vi "DAQ-node.vi"() -> ()   [LabVIEW 2024]
uses:
  CTRsample/Control/StreamTypeDef.ctl
  CTRsample/Control/streamIO_states.ctl
  <vilib>/Platform/TimedLoop/XDataNode/timing_clust.ctl
  <vilib>/Platform/TimedLoop/XDataNode/nitl_modes.ctl
  <vilib>/Platform/TimedLoop/XDataNode/wakeup.ctl
  <vilib>/DAQmx/read.llb/DAQmx Read (Analog 2D DBL NChan NSamp).vi
  <vilib>/DAQmx/create/channels.llb/DAQmx Create Channel (AI-Voltage-Basic).vi
  <vilib>/DAQmx/configure/timing.llb/DAQmx Timing (Sample Clock).vi
  Control/state.vi
  <vilib>/DAQmx/miscellaneous.llb/DAQmx Fill In Error Info.vi
  <vilib>/platform/TimedLoop/XDataNode/XDataNode.xnode
  <vilib>/Platform/TimedLoop/XDataNode/XDNodeRunTimeDep.lvlib
panel:
  out "dT":i64
  out "Clock (ms)":cluster{i64, "Period":i64}(graph)
  out "error out":errorcluster
  in  "StreamTypeDef":T1
  out "Waveform Chart":dbl[][](graph)
  in  "stop":bool
  in  "error in":errorcluster
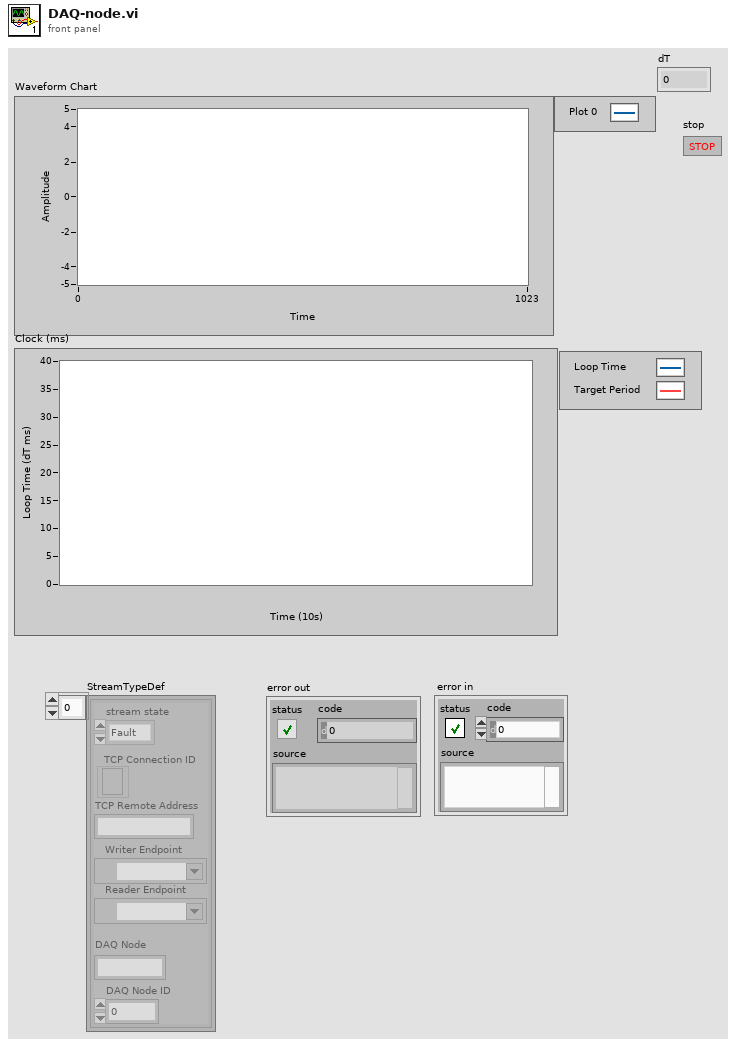
[diagram p1: front panel]
types:
  T1 = typedef "StreamTypeDef.ctl" = cluster{"stream state":T2, "TCP Remote Address":string, "TCP Connection ID":refnum<k5>, "DAQ Node":string, "DAQ Node ID":i32, "Writer Endpoint":refnum<k21>, "Reader Endpoint":refnum<k21>}[]
  T2 = typedef "streamIO_states.ctl" = enum16{"Fault", "Initilize", "Stream", "Close"}
  T3 = cluster{"StreamTypeDef[0]":cluster{"stream state":T2, "TCP Remote Address":string, "TCP Connection ID":refnum<k5>, "DAQ Node":string, "DAQ Node ID":i32, "Writer Endpoint":refnum<k21>, "Reader Endpoint":refnum<k21>}}
  T4 = cluster{"stream state":T2, "TCP Remote Address":string, "TCP Connection ID":refnum<k5>, "DAQ Node":string, "DAQ Node ID":i32, "Writer Endpoint":refnum<k21>, "Reader Endpoint":refnum<k21>}
  T5 = typedef "XDNodeRunTimeDep.lvlib/timing_clust.ctl" = cluster{"Expected End [f-1]":u64, "Actual End [f-1]":u64, "Finished Late? [f-1]":bool, "Expected End [i-1]":u64, "Actual End [i-1]":u64, "Finished Late? [i-1]":bool, "Expected Start [i]":u64, "Actual Start [i]":u64, "Expected Start [f]":u64, "Actual Start [f]":u64, "Source Name":string, "Structure Name":string, "Period":i64, "Deadline":i64, "Offset":i64, "Start":i64, "Priority":i32, "Timeout":i32, "Mode":T6, "Wakeup Reason":T7, "Error":errorcluster, "Source Type":string, "Secondary Source Type":string, "Global End Time":u64, "Global Start Time":u64, "Frame Duration":u64, "Iteration Duration":u64, "Assigned CPU":i32, "I/O Scan Engine Mode":u32}
  T6 = typedef "XDNodeRunTimeDep.lvlib/nitl_modes.ctl" = enum32{"No Change", "Process missed periods, maintain original phase", "Discard missed periods, maintain original phase", "Process missed periods, ignore original phase", "Discard missed periods, ignore original phase"}
  T7 = typedef "XDNodeRunTimeDep.lvlib/wakeup.ctl" = enum32{"Normal", "Aborted", "Asynchronous wakeup", "Timing source error", "Timed loop error", "Timeout"}
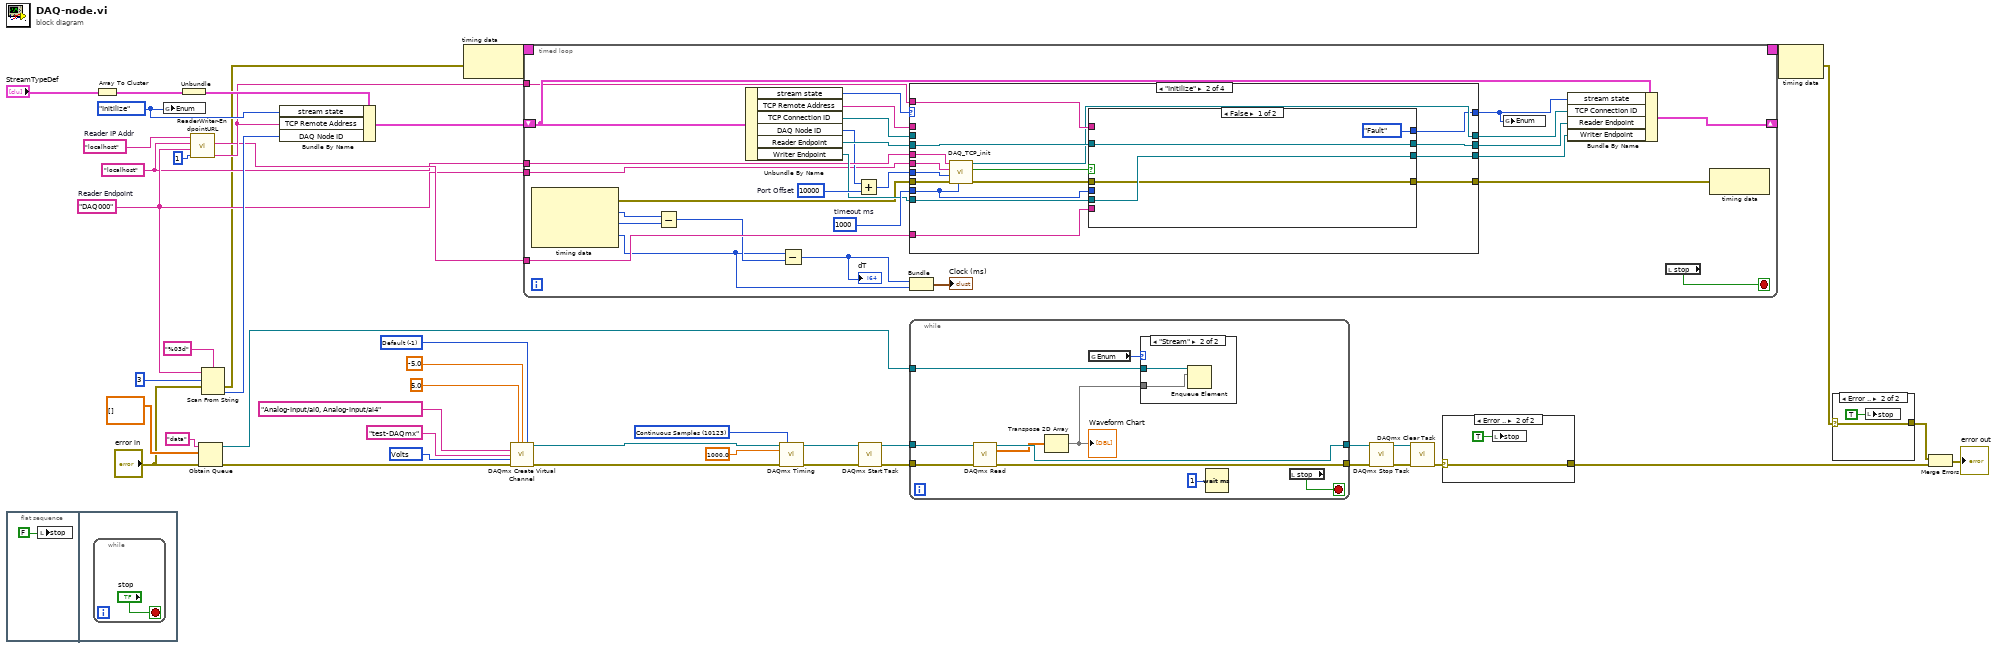
[diagram p0: block diagram]
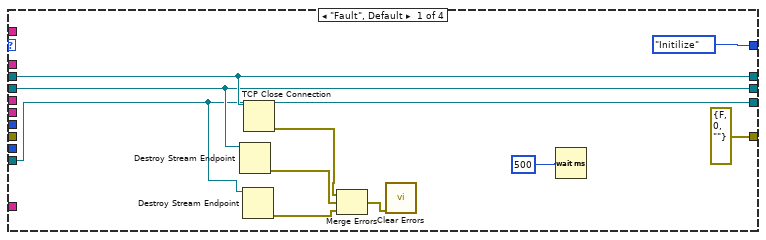
[diagram p4: hidden frame]
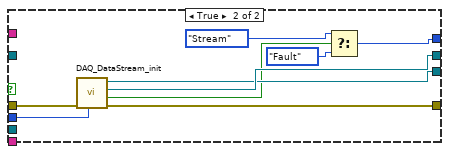
[diagram p5: hidden frame]
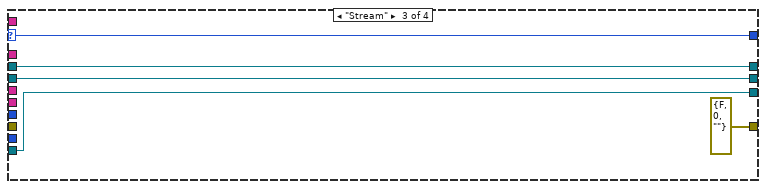
[diagram p6: hidden frame]
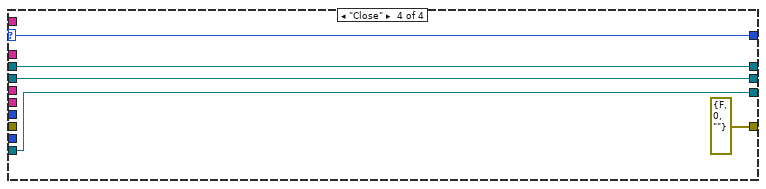
[diagram p7: hidden frame]
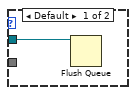
[diagram p8: hidden frame]
diagram:
  w11 = "localhost" ("DAQ IR Addr")
  w15 = "localhost"  # Reader IP Addr
  w12 = "DAQ000"  # Reader Endpoint
  w20 = streamIO_states."Initilize" ("Enum")
  w35 = 10123 items=["Finite Samples"=10178, "Continuous Samples"=10123, "Hardware Timed Single Point"=12522] ("sample mode")
  w38 = 10348 items=["Volts"=10348, "From Custom Scale"=10065] ("units")
  w43 = -1 items=["Default"=-1, "RSE"=10083, "NRSE"=10078, "Differential"=10106, "Pseudodifferential"=12529] ("input terminal configuration")
  n1 = flat-sequence {
    frame #0 {
      n2 = local write "stop"(FALSE ("stop")) -> ()
    }
    frame #1 {
      n3 = while {
        stop <- "stop" stop-if-true
      }
    }
  }
  n4 = Array To Cluster(array="StreamTypeDef") -> (cluster=w23:T3)
  n5 = global write "state.vi" "Enum"(w20) -> ()
  n6 = Unbundle(w23) -> ("StreamTypeDef[0]"=w22:T4)
  n7 = call "ReaderWriter-EndpointURL.vi"("CTR ID #"=1 ("DAQ ID #"), "DAQ Endpoint"=w12, "CTR IR Addr"=w11, "DAQ IP Addr"=w15) -> ("DAQ Endpoint"=w14:string, "CTR URL"=w13:string)  [unwired: 4 in, 2 out]
  n8 = Obtain Queue(name (unnamed)="data", element data type=dbl[][] [] ("data"), error in (no error)="error in") -> (queue out=w25:refnum<queue>, error out=w8:errorcluster)  [unwired: 2 in, 1 out]
  n9 = Scan From String(format string="%03d", input string=w12, initial scan location=u32 3, error in="error in") -> (error out=w6:errorcluster, output 1=w17:i32)  [unwired: 1 in, 2 out]
  n10 = Bundle By Name(cluster=w22, "stream state"=w20, "TCP Remote Address"=w14, "DAQ Node ID"=w17) -> (w21:T4)
  n11 = node-c288(w6) -> (w10:T5)
  n12 = call-poly <vilib>:"DAQmx Create Virtual Channel.vi"("maximum value"=5.0, "minimum value"=-5.0, "input terminal configuration"=w43, "physical channels"=tag "Analog-Input/ai0, Analog-Input/ai4", "name to assign"="test-DAQmx", "units"=w38, "error in"=w8) -> ("task out"=w34:refnum<k21>, "error out"=w28:errorcluster)  [unwired: 7 in]
  n13 = timed-loop {
    shift-right: [w73] -> _
    shift-left: w21 -> [w72]
    tunnel: w11 -> [w62]
    tunnel: w12 -> [w60]
    tunnel: w14 -> [w59]
    tunnel: w13 -> [w58]
    timing: w10 -> [_]
    timing-out: [_] -> w9
    stop <- w75 stop-if-true
    w66 = 1000  # timeout ms
    w68 = 10000  # Port Offset
    n14 = node-c288() -> (w55:errorcluster, w52:i64, w51:i64, w49:i64)  [unwired: 1 in]
    n15 = Subtract(x=w52, y=w51) -> (x-y=w50:i64)
    n16 = Unbundle By Name(w72) -> ("stream state"=w74:T2, "TCP Remote Address"=w70:string, "TCP Connection ID"=w69:refnum<k5>, "DAQ Node ID"=w61:i32, "Reader Endpoint"=w65:refnum<k21>, "Writer Endpoint"=w64:refnum<k21>)
    n17 = Subtract(x=w49, y=w50) -> (x-y=w48:i64)
    "dT" <- w48
    n18 = Add(x=w61, y=w68) -> (x+y=w67:i32)
    n19 = case shown="\"Initilize\"" w74 {
      selector: w74 -> [_ _ w127 w132]
      tunnel: [streamIO_states."Initilize" ("Enum") w94 w127 w132] -> w71
      tunnel: w70 -> [_ _ _ _]
      tunnel: w69 -> [w88 _ w125 w131]
      tunnel: w67 -> [_ w103 _ _]
      tunnel: w66 -> [_ w100 _ _]
      tunnel: w65 -> [w87 w104 w124 w130]
      tunnel: w64 -> [w86 w105 w123 w129]
      tunnel: [w88 w99 w125 w131] -> w63
      tunnel: w62 -> [_ w98 _ _]
      tunnel: w60 -> [_ w97 _ _]
      tunnel: w59 -> [_ w109 _ _]
      tunnel: w58 -> [_ w108 _ _]
      tunnel: [w86 w107 w123 w129] -> w56
      tunnel: [w87 w106 w124 w130] -> w57
      tunnel: [errorcluster {"status"=FALSE, "code"=0, "source"=""} ("error out") w96 errorcluster {"status"=FALSE, "code"=0, "source"=""} ("error out") errorcluster {"status"=FALSE, "code"=0, "source"=""} ("error out")] -> w54
      tunnel: w55 -> [_ w95 _ _]
      frame "Fault", Default {
        n20 = Destroy Stream Endpoint(11:w87) -> (0:w91:errorcluster)  [unwired: 1 in]
        n21 = Destroy Stream Endpoint(11:w86) -> (0:w92:errorcluster)  [unwired: 1 in]
        n22 = TCP Close Connection(connection ID=w88) -> (error out=w90:errorcluster)  [unwired: 2 in, 1 out]
        n23 = Merge Errors(w90, w91, w92) -> (w89:errorcluster)
        n24 = call <vilib>:"Clear Errors.vi"("error in (no error)"=w89) -> ()  [unwired: 5 in, 2 out]
        n25 = Wait (ms)(milliseconds to wait=u32 500) -> ()  [unwired: 1 out]
      }
      frame "Initilize" {
        n26 = call "DAQ_TCP_init.vi"("timeout ms (60000)"=w100, "error in"=w95, "remote port or service name"=w103, "DAQ refDes"=w97, "address"=w98) -> ("error out"=w101:errorcluster, "TCP Success?"=w102:bool, "connection ID"=w99:refnum<k5>)  [unwired: 4 in]
        n27 = case shown="False" w102 {
          tunnel: w100 -> [_ w118]
          tunnel: [w113 w120] -> w107
          tunnel: [w112 w121] -> w106
          tunnel: w109 -> [_ _]
          tunnel: w108 -> [_ _]
          tunnel: w105 -> [w113 _]
          tunnel: w104 -> [w112 _]
          tunnel: w101 -> [w111 w122]
          tunnel: [w111 w119] -> w96
          tunnel: [streamIO_states."Fault" ("stream state") w115] -> w94
          frame False {
          }
          frame True {
            n28 = call "DAQ_DataStream_init.vi"("timeout ms"=w118, "error in"=w122) -> ("error out"=w119:errorcluster, "Streams Started?"=w114:bool, "reader endpoint"=w121:refnum<k21>, "writer endpoint"=w120:refnum<k21>)  [unwired: 6 in]
            n29 = Select(t=streamIO_states."Stream" ("stream state"), s=w114, f=streamIO_states."Fault" ("stream state")) -> (s? t:f=w115:T2)
          }
        }
      }
      frame "Stream" {
      }
      frame "Close" {
      }
    }
    n30 = Bundle(w48, "Period"=w49) -> (→"Clock (ms)":cluster{i64, "Period":i64})  [unwired: 1 in]
    n31 = global write "state.vi" "Enum"(w71) -> ()
    n32 = Bundle By Name(cluster=w72, "stream state"=w71, "TCP Connection ID"=w63, "Reader Endpoint"=w57, "Writer Endpoint"=w56) -> (w73:T4)
    n33 = local read "stop"() -> (w75:bool)
    n34 = node-c288(w54) -> ()  [unwired: 1 out]
  }
  n35 = call-poly <vilib>:"DAQmx Timing.vi"("task/channels in"=w34, "sample mode"=w35, "rate"=1000.0, "error in"=w28) -> ("task out"=w36:refnum<k21>, "error out"=w37:errorcluster)  [unwired: 10 in]
  n36 = call <vilib>:"DAQmx Start Task.vi"("task/channels in"=w36, "error in"=w37) -> ("task out"=w32:refnum<k21>, "error out"=w31:errorcluster)  [unwired: 12 in]
  n37 = while {
    tunnel: w32 -> [w141]
    tunnel: w31 -> [w140]
    tunnel: [w139] -> w30
    tunnel: [w138] -> w29
    tunnel: w25 -> [w135]
    stop <- w133 stop-if-true
    n38 = call-poly <vilib>:"DAQmx Read.vi"("task/channels in"=w141, "error in"=w140) -> ("task out"=w138:refnum<k21>, "data"=w137:dbl[][], "error out"=w139:errorcluster)  [unwired: 11 in]
    n39 = Transpose 2D Array(2D array=w137) -> (transposed array=w136:dbl[][])
    "Waveform Chart" <- w136
    n40 = global read "state.vi" "Enum"() -> (w134:T2)
    n41 = case shown="\"Stream\"" w134 {
      tunnel: w136 -> [_ w145]
      tunnel: w135 -> [w143 w144]
      frame Default {
        n42 = Flush Queue(queue=w143) -> ()  [unwired: 1 in, 3 out]
      }
      frame "Stream" {
        n43 = Enqueue Element(queue=w144, element=w145) -> ()  [unwired: 2 in, 3 out]
      }
    }
    n44 = Wait (ms)(milliseconds to wait=u32 1) -> ()  [unwired: 1 out]
    n45 = local read "stop"() -> (w133:bool)
  }
  n46 = call <vilib>:"DAQmx Stop Task.vi"("task/channels in"=w29, "error in"=w30) -> ("task out"=w45:refnum<k21>, "error out"=w44:errorcluster)  [unwired: 12 in]
  n47 = call <vilib>:"DAQmx Clear Task.vi"("task in"=w45, "error in"=w44) -> ("error out"=w5:errorcluster)  [unwired: 13 in]
  n48 = case shown="Error .." w5 {
    selector: w5 -> [w146 w147]
    tunnel: [w146 w147] -> w3
    frame No Error {
    }
    frame Error {
      n49 = local write "stop"(TRUE ("stop")) -> ()
    }
  }
  n50 = node-c288(w9) -> (w4:errorcluster)
  n51 = case shown="Error .." w4 {
    selector: w4 -> [w149 w150]
    tunnel: [w149 w150] -> w2
    frame No Error {
    }
    frame Error {
      n52 = local write "stop"(TRUE ("stop")) -> ()
    }
  }
  n53 = Merge Errors(w2, w3) -> (→"error out":errorcluster)
